vi "Obtain Broadcast Events.vi"(8 "error in (no error)":errorcluster, 10 "Create New? (F)":bool) -> (0 "error out":errorcluster, 2 "Serial-Com-Module Broadcast Events":T1)   [LabVIEW 2022 SP3, in "Serial-Com-Module.lvlib"]
doc: "This VI Obtains/Creates the Broadcast events that will be used for other modules to register to receive messages from the module that owns this VI.\n\n<b>NOTE</b>: The contents of this VI are automatically generated and modified by the <b>Tools > Delacor > DQMH</b> utilities. Consider using those utilities instead of making your own modifications to this VI.\n_____\nBased on DQMH Project Template 6.1.0.94."
uses:
  Serial-Com-Module.lvlib
  Broadcast Events--cluster.ctl
  Did Init Argument--cluster.ctl
  Status Updated Argument--cluster.ctl
  Error Reported Argument--cluster.ctl
  Stop Argument--cluster.ctl
  Get Module Execution Status Argument--cluster.ctl
  Init Serial (Reply Payload)--cluster.ctl
  Open Port (Reply Payload)--cluster.ctl
  Close Port (Reply Payload)--cluster.ctl
panel:
  # "NOTE: The contents of this VI are automatically generated and modified by the Tools > Delacor > DQMH utilities. Consider using those utilities instead of making your own modifications to this VI."
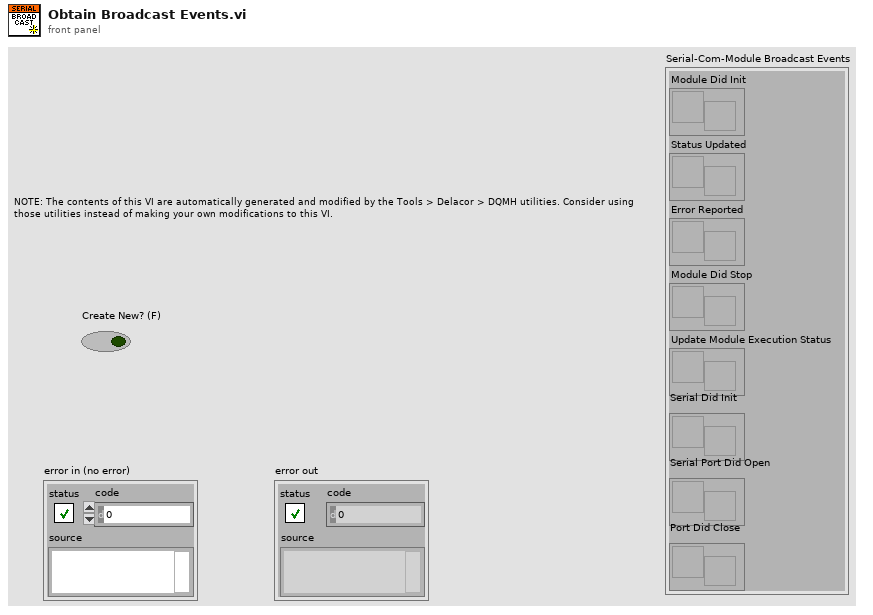
[diagram p1: front panel]
types:
  T1 = typedef "Serial-Com-Module.lvlib/Broadcast Events--cluster.ctl" = cluster{"Module Did Init":refnum<user-event>, "Status Updated":refnum<user-event>, "Error Reported":refnum<user-event>, "Module Did Stop":refnum<user-event>, "Update Module Execution Status":refnum<user-event>, "Serial Did Init":refnum<user-event>, "Serial Port Did Open":refnum<user-event>, "Port Did Close":refnum<user-event>}
  T2 = typedef "Serial-Com-Module.lvlib/Close Port (Reply Payload)--cluster.ctl" = cluster{"error":errorcluster}
  T3 = typedef "Serial-Com-Module.lvlib/Open Port (Reply Payload)--cluster.ctl" = cluster{"error":errorcluster}
  T4 = typedef "Serial-Com-Module.lvlib/Init Serial (Reply Payload)--cluster.ctl" = cluster{"error":errorcluster}
  T5 = typedef "Serial-Com-Module.lvlib/Get Module Execution Status Argument--cluster.ctl" = cluster{"Module ID":i32, "Running?":bool}
  T6 = typedef "Serial-Com-Module.lvlib/Stop Argument--cluster.ctl" = cluster{"Module ID":i32, "Origin":string, "Exit via Stop Module Req?":bool, "Wait for Module to stop?":bool}
  T7 = typedef "Serial-Com-Module.lvlib/Error Reported Argument--cluster.ctl" = cluster{"Error":errorcluster, "Additional Information":string, "Module ID":i32, "Module Name":string}
  T8 = typedef "Serial-Com-Module.lvlib/Status Updated Argument--cluster.ctl" = cluster{"Status":string, "Module ID":i32}
  T9 = typedef "Serial-Com-Module.lvlib/Did Init Argument--cluster.ctl" = cluster{"Init?":bool, "Info":string, "Module ID":i32}
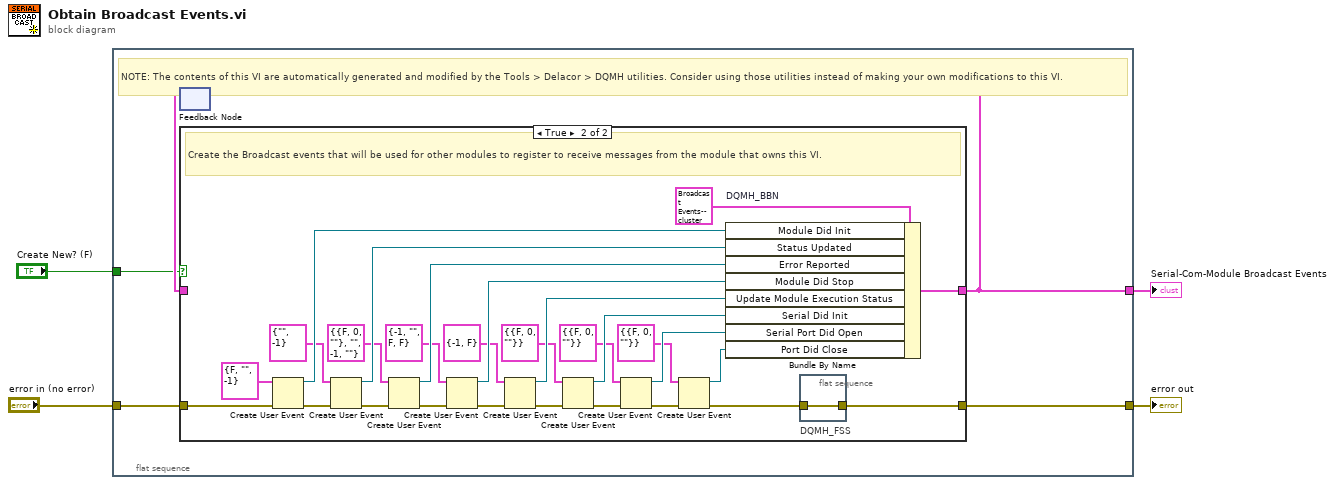
[diagram p0: block diagram]
diagram:
  n1 = flat-sequence {
    tunnel: [w9] -> w4
    tunnel: "error in (no error)" -> [w8]
    tunnel: [w6] -> w2
    tunnel: "Create New? (F)" -> [w5]
    frame #0 {
      # "NOTE: The contents of this VI are automatically generated and modified by the Tools > Delacor > DQMH utilities. Consider using those utilities instead of making your own modifications to this VI."
      n2 = feedback #1() -> (w7:T1)  [unwired: 1 in]
      n3 = case shown="True" w5 {
        tunnel: [w10 w24] -> w9
        tunnel: w8 -> [w10 w39]
        tunnel: [w11 w36] -> w6
        tunnel: w7 -> [w11 _]
        frame False {
          # "Obtain the Broadcast events that were created in a previous call to this VI."
        }
        frame True {
          # "Create the Broadcast events that will be used for other modules to register to receive messages from the module that owns this VI."
          n4 = Create User Event(user event datatype=T9 {"Init?"=FALSE, "Info"="", "Module ID"=-1} ("Did Init Argument"), error in=w39) -> (user event=w37:refnum<user-event>, error out=w34:errorcluster)
          n5 = Create User Event(user event datatype=T8 {"Status"="", "Module ID"=-1} ("Status Updated Argument"), error in=w34) -> (user event=w31:refnum<user-event>, error out=w33:errorcluster)
          n6 = Create User Event(user event datatype=T7 {"Error"={"status"=FALSE, "code"=0, "source"=""}, "Additional Information"="", "Module ID"=-1, "Module Name"=""} ("Error Reported Argument"), error in=w33) -> (user event=w28:refnum<user-event>, error out=w30:errorcluster)
          n7 = Create User Event(user event datatype=T6 {"Module ID"=-1, "Origin"="", "Exit via Stop Module Req?"=FALSE, "Wait for Module to stop?"=FALSE} ("Stop Argument"), error in=w30) -> (user event=w26:refnum<user-event>, error out=w25:errorcluster)
          n8 = Create User Event(user event datatype=T5 {"Module ID"=-1, "Running?"=FALSE} ("Get Module Execution Status Argument"), error in=w25) -> (user event=w22:refnum<user-event>, error out=w23:errorcluster)
          n9 = Create User Event(user event datatype=T4 {"error"={"status"=FALSE, "code"=0, "source"=""}} ("Init Serial (Reply Payload)"), error in=w23) -> (user event=w19:refnum<user-event>, error out=w20:errorcluster)
          n10 = Create User Event(user event datatype=T3 {"error"={"status"=FALSE, "code"=0, "source"=""}} ("Open Port (Reply Payload)"), error in=w20) -> (user event=w16:refnum<user-event>, error out=w17:errorcluster)
          n11 = Create User Event(user event datatype=T2 {"error"={"status"=FALSE, "code"=0, "source"=""}} ("Close Port (Reply Payload)"), error in=w17) -> (user event=w13:refnum<user-event>, error out=w14:errorcluster)
          n12 = Bundle By Name "DQMH_BBN"(cluster=T1 {"Module Did Init"=refnum, "Status Updated"=refnum, "Error Reported"=refnum, "Module Did Stop"=refnum, "Update Module Execution Status"=refnum, "Serial Did Init"=refnum, "Serial Port Did Open"=refnum, "Port Did Close"=refnum} ("output cluster"), "Module Did Init"=w37, "Status Updated"=w31, "Error Reported"=w28, "Module Did Stop"=w26, "Update Module Execution Status"=w22, "Serial Did Init"=w19, "Serial Port Did Open"=w16, "Port Did Close"=w13) -> (w36:T1)
          n13 = flat-sequence "DQMH_FSS" {
            tunnel: w14 -> [w40]
            tunnel: [w40] -> w24
            frame #0 {
            }
          }
        }
      }
      n14 = feedback-in #1(w6) -> ()
    }
  }
  "Serial-Com-Module Broadcast Events" <- w2
  "error out" <- w4
